vi "quote and escape json string 2.vi"(11 "base string":string) -> (3 "String out":string)   [LabVIEW 2015, in "JSONtext.lvlib"]
uses:
  JSONtext.lvlib
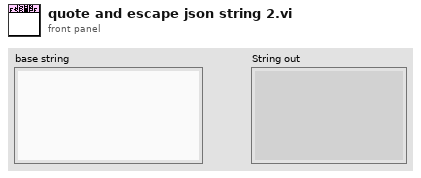
[diagram p1: front panel]
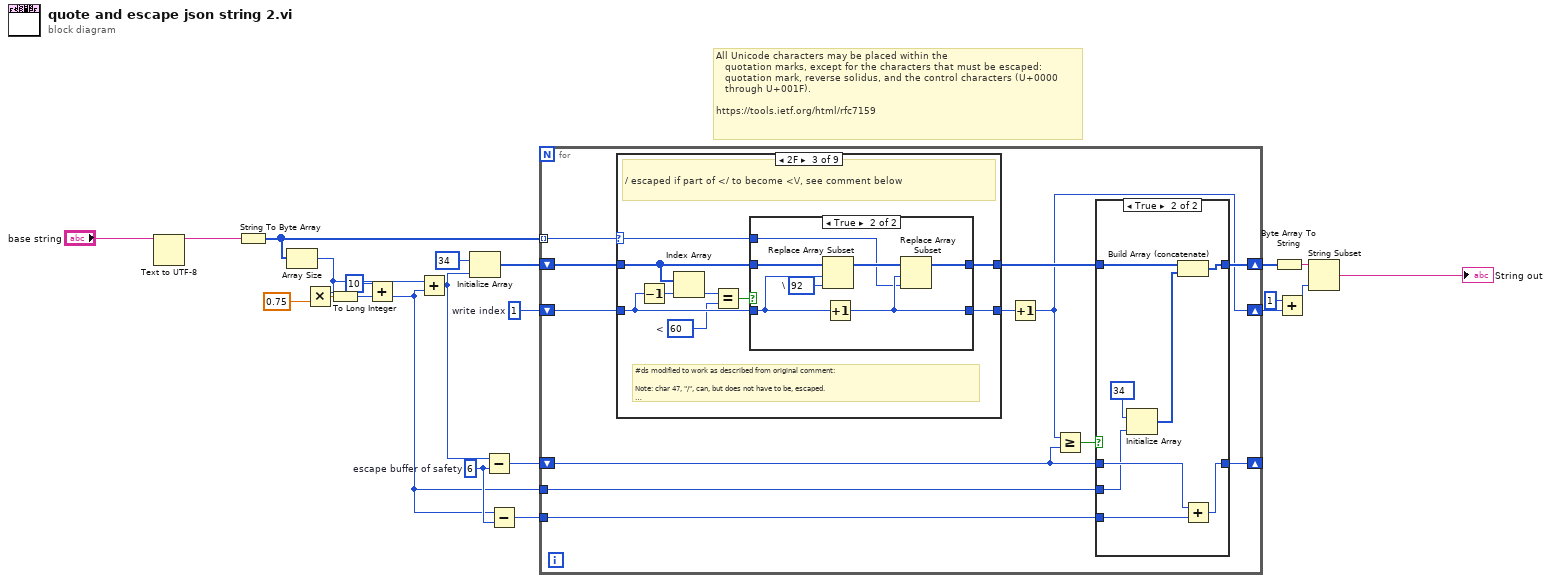
[diagram p0: block diagram]
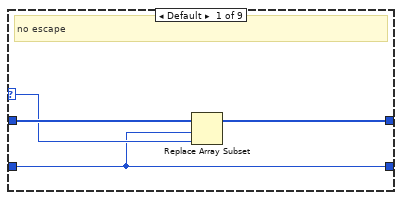
[diagram p3: hidden frame]
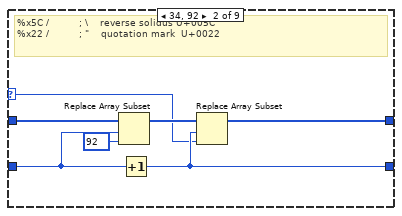
[diagram p4: hidden frame]
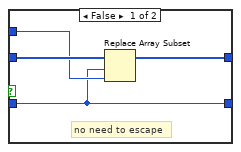
[diagram p5: hidden frame]
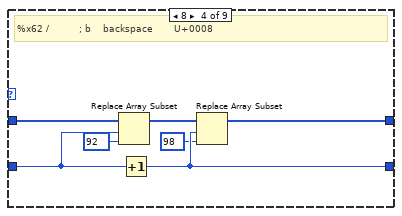
[diagram p6: hidden frame]
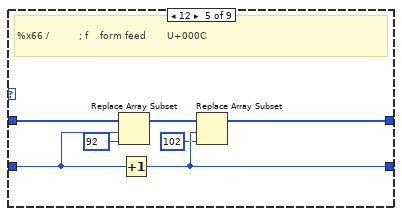
[diagram p7: hidden frame]
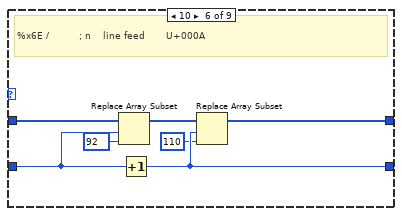
[diagram p8: hidden frame]
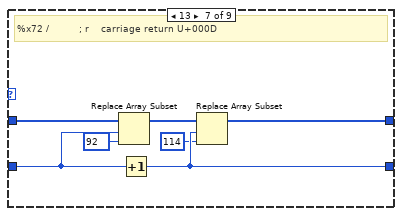
[diagram p9: hidden frame]
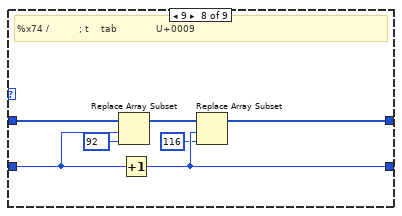
[diagram p10: hidden frame]
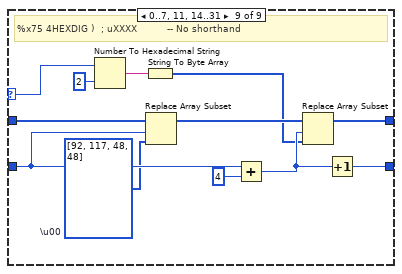
[diagram p11: hidden frame]
diagram:
  w8 = 6  # escape buffer of safety
  w20 = 1  # write index
  # "All Unicode characters may be placed within the\n   quotation marks, except for the characters that must be escaped:\n   quotation mark, reverse solidus, and the control characters (U+0000\n   through U+001F).\n\nhttps://tools.ietf.org/html/rfc7159"
  n1 = Text to UTF-8(11:"base string") -> (3:w1:string)  [unwired: 2 in, 1 out]
  n2 = String To Byte Array(string=w1) -> (unsigned byte array=w14:u8[])
  n3 = Array Size(array=w14) -> (size(s)=w12:i32)
  n4 = Multiply(x=w12, y=0.75) -> (x*y=w15:dbl)
  n5 = To Long Integer(number=w15) -> (32bit integer=w9:i32)
  n6 = Add(x=10, y=w9) -> (x+y=w5:i32)
  n7 = Add(x=w12, y=w5) -> (x+y=w11:i32)
  n8 = Initialize Array(u8 34, w11) -> (w17:u8[])
  n9 = Subtract(x=w11, y=w8) -> (x-y=w10:i32)
  n10 = Subtract(x=w5, y=w8) -> (x-y=w7:i32)
  n11 = for {
    shift-right: [w31] -> w19
    shift-left: w17 -> [w34]
    shift-right: [w24] -> w13
    shift-left: w20 -> [w33]
    tunnel: w14 -> [w32] mode=indexing
    shift-right: [w28] -> _
    shift-left: w10 -> [w27]
    tunnel: w5 -> [w26]
    tunnel: w7 -> [w25]
    n12 = case shown="2F" w32 {
      selector: w32 -> [w46 w50 w62 _ _ _ _ _ w119]
      tunnel: w34 -> [w48 w55 w61 w82 w89 w96 w103 w110 w122]
      tunnel: [w47 w52 w64 w79 w86 w93 w100 w107 w121] -> w30
      tunnel: w33 -> [w45 w53 w60 w80 w87 w94 w101 w108 w120]
      tunnel: [w45 w51 w63 w78 w85 w92 w99 w106 w111] -> w29
      frame Default {
        # "no escape"
        n13 = Replace Array Subset(array=w48, new element=w46, index=w45) -> (w47:u8[])
      }
      frame 34, 92 {
        # "%x5C /          ; \\    reverse solidus U+005C\n%x22 /          ; \"    quotation mark  U+0022"
        n14 = Replace Array Subset(array=w55, new element=u8 92 ("new element/subarray"), index=w53) -> (w54:u8[])
        n15 = Increment(x=w53) -> (x+1=w51:i32)
        n16 = Replace Array Subset(array=w54, new element=w50, index=w51) -> (w52:u8[])
      }
      frame 47 {
        w56 = u8 60  # <
        # "#ds modified to work as described from original comment:\n\nNote: char 47, \"/\", can, but does not have to be, escaped.\n\nSee Errata 3159 for RFC4627.   -- JDP\n\nSo we only escape \"/\" if it is part of \"</\", as this is\nthe case that needs escaping to put JSON in a\n<script>...</script> HTML tag  -- JDP Nov, 2014"
        # "/ escaped if part of </ to become <\\/, see comment below"
        n17 = Decrement(x=w60) -> (x-1=w59:i32)
        n18 = Index Array(array=w61, index=w59) -> (element=w58:u8)
        n19 = Equal?(x=w58, y=w56) -> (x = y?=w57:bool)
        n20 = case shown="True" w57 {
          tunnel: [w67 w74] -> w64
          tunnel: [w65 w73] -> w63
          tunnel: w62 -> [w66 w72]
          tunnel: w61 -> [w68 w71]
          tunnel: w60 -> [w65 w70]
          frame False {
            # "no need to escape"
            n21 = Replace Array Subset(array=w68, new element=w66, index=w65) -> (w67:u8[])
          }
          frame True {
            w69 = u8 92  # \
            n22 = Replace Array Subset(array=w71, new element=w69, index=w70) -> (w75:u8[])
            n23 = Increment(x=w70) -> (x+1=w73:i32)
            n24 = Replace Array Subset(array=w75, new element=w72, index=w73) -> (w74:u8[])
          }
        }
      }
      frame 8 {
        # "%x62 /          ; b    backspace       U+0008"
        n25 = Replace Array Subset(array=w82, new element=u8 92 ("new element/subarray"), index=w80) -> (w81:u8[])
        n26 = Increment(x=w80) -> (x+1=w78:i32)
        n27 = Replace Array Subset(array=w81, new element=u8 98 ("new element/subarray"), index=w78) -> (w79:u8[])
      }
      frame 12 {
        # "%x66 /          ; f    form feed       U+000C"
        n28 = Replace Array Subset(array=w89, new element=u8 92 ("new element/subarray"), index=w87) -> (w88:u8[])
        n29 = Increment(x=w87) -> (x+1=w85:i32)
        n30 = Replace Array Subset(array=w88, new element=u8 102 ("new element/subarray"), index=w85) -> (w86:u8[])
      }
      frame 10 {
        # "%x6E /          ; n    line feed       U+000A"
        n31 = Replace Array Subset(array=w96, new element=u8 92 ("new element/subarray"), index=w94) -> (w95:u8[])
        n32 = Increment(x=w94) -> (x+1=w92:i32)
        n33 = Replace Array Subset(array=w95, new element=u8 110 ("new element/subarray"), index=w92) -> (w93:u8[])
      }
      frame 13 {
        # "%x72 /          ; r    carriage return U+000D"
        n34 = Replace Array Subset(array=w103, new element=u8 92 ("new element/subarray"), index=w101) -> (w102:u8[])
        n35 = Increment(x=w101) -> (x+1=w99:i32)
        n36 = Replace Array Subset(array=w102, new element=u8 114 ("new element/subarray"), index=w99) -> (w100:u8[])
      }
      frame 9 {
        # "%x74 /          ; t    tab             U+0009"
        n37 = Replace Array Subset(array=w110, new element=u8 92 ("new element/subarray"), index=w108) -> (w109:u8[])
        n38 = Increment(x=w108) -> (x+1=w106:i32)
        n39 = Replace Array Subset(array=w109, new element=u8 116 ("new element/subarray"), index=w106) -> (w107:u8[])
      }
      frame 0..7, 11, 14..31 {
        w112 = u8[] [92, 117, 48, 48]  # \u00
        # "%x75 4HEXDIG )  ; uXXXX          -- No shorthand"
        n40 = Number To Hexadecimal String(1:i16 2 ("width (-)"), 2:w119) -> (0:w114:string)
        n41 = String To Byte Array(string=w114) -> (unsigned byte array=w116:u8[])
        n42 = Replace Array Subset(array=w122, new element=w112, index=w120) -> (w118:u8[])
        n43 = Add(x=w120, y=4) -> (x+y=w117:i32)
        n44 = Replace Array Subset(array=w118, new element=w116, index=w117) -> (w121:u8[])
        n45 = Increment(x=w117) -> (x+1=w111:i32)
      }
    }
    n46 = Increment(x=w29) -> (x+1=w24:i32)
    n47 = Greater Or Equal?(x=w24, y=w27) -> (x >= y?=w23:bool)
    n48 = case shown="True" w23 {
      tunnel: [w36 w39] -> w31
      tunnel: w30 -> [w36 w40]
      tunnel: [w35 w42] -> w28
      tunnel: w27 -> [w35 w43]
      tunnel: w26 -> [_ w41]
      tunnel: w25 -> [_ w44]
      frame False {
      }
      frame True {
        n49 = Initialize Array(u8 34, w41) -> (w38:u8[])
        n50 = Build Array (concatenate)(w40, w38) -> (w39:u8[])
        n51 = Add(x=w43, y=w44) -> (x+y=w42:i32)
      }
    }
  }
  n52 = Byte Array To String(unsigned byte array=w19) -> (string=w21:string)
  n53 = Add(x=1, y=w13) -> (x+y=w6:i32)
  n54 = String Subset(string=w21, length (rest)=w6) -> (substring=→"String out":string)  [unwired: 1 in]
